vi "Read Config VI.vi"(8 "error in (no error)":errorcluster, 11 "CsvReportPlugin in":refnum<class "CsvReportPlugin.lvclass">) -> (0 "error out":errorcluster, 2 "VI Refnum":refnum<vi>, 3 "CsvReportPlugin out":refnum<class "CsvReportPlugin.lvclass">)   [LabVIEW 2015, in "CsvReportPlugin.lvclass"]
uses:
  CsvReportPlugin.lvclass
  Config VI.vi
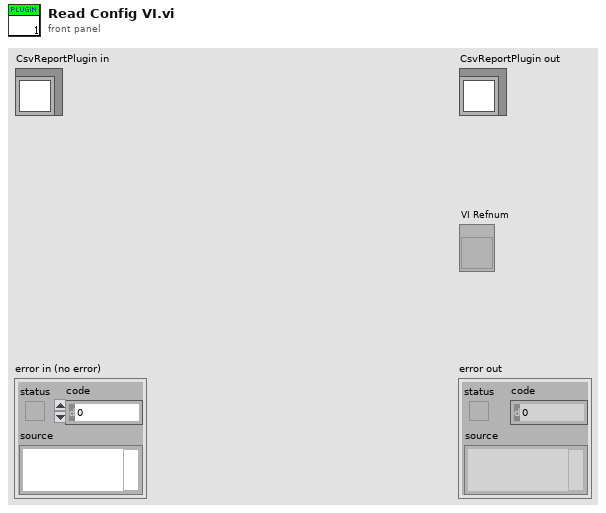
[diagram p1: front panel]
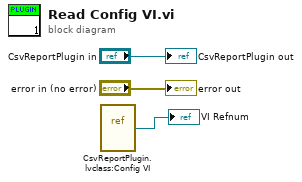
[diagram p0: block diagram]
diagram:
  n1 = vi-ref "CsvReportPlugin.lvclass:Config VI.vi"() -> (→"VI Refnum":refnum<vi>)
  "error out" <- "error in (no error)"
  "CsvReportPlugin out" <- "CsvReportPlugin in"
